vi "VarValueEventCallabck.vi"(4 "User Parameter":variant, 5 "Event Data":cluster{"sender":refnum<k24>, "e":refnum<k24>}, 6 "Control Ref":refnum<k24>, 7 "Event Common Data":T1) -> ()   [LabVIEW 2022 SP3]
uses:
  C:/Software Repos/shared components/SECSGEM/DotNet20EqApp/GemEqApp/SecsPort.dll
  Software Repos/shared components/SECSGEM/DotNet20EqApp/GemEqApp/SecsPort.dll
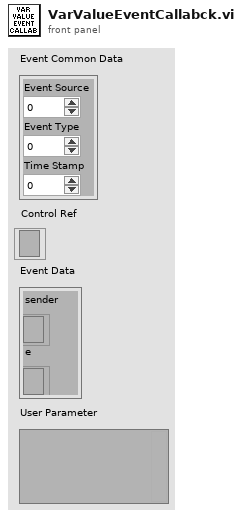
[diagram p1: front panel]
types:
  T1 = cluster{"Event Source":i32, "Event Type":u32, "Time Stamp":u32}
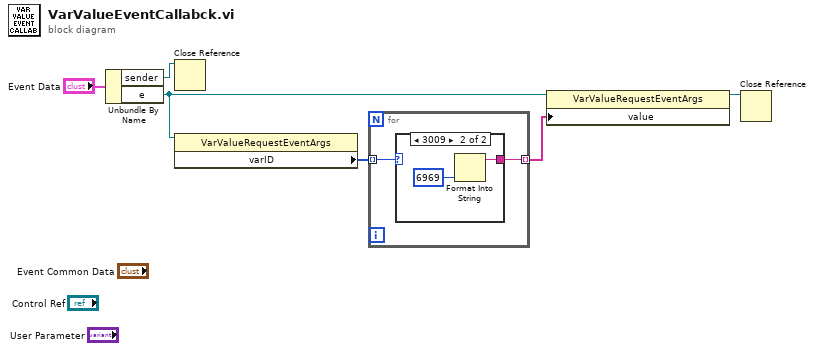
[diagram p0: block diagram]
diagram:
  n1 = Unbundle By Name("Event Data") -> ("sender"=w1:refnum<k24>, "e"=w3:refnum<k24>)
  n2 = Close Reference(reference=w1) -> ()  [unwired: 1 in, 1 out]
  n3 = property class="VarValueRequestEventArgs"(reference=w3) -> ("varID"=w5:i32[])  [unwired: 1 in, 2 out]
  n4 = for {
    tunnel: w5 -> [w8] mode=indexing
    tunnel: [w7] -> w4 mode=indexing
    n5 = case shown="3009" w8 {
      tunnel: [_ w9] -> w7
      frame Default {
      }
      frame 3009 {
        n6 = Format Into String(6969) -> (resulting string=w9:string)  [unwired: 3 in, 1 out]
      }
    }
  }
  n7 = property class="VarValueRequestEventArgs"(reference=w3, "value"=w4) -> (reference out=w2:refnum<k24>)  [unwired: 1 in, 1 out]
  n8 = Close Reference(reference=w2) -> ()  [unwired: 1 in, 1 out]
